vi "Absturz.vi"() -> ()   [LabVIEW 2020]
uses:
  <vilib>/xnet/xnet.llb/XNET Frame Type CAN.ctl
  <vilib>/xnet/xnet.llb/XNET Frame CAN.ctl
panel:
  out "I64":i64[](array[numeric])
  out "U64":u64[](array[numeric])
  in  "Numerisch":i32
  out "identifier":u32
  in  "Index":i32
  in  "CAN data 2":T1[](array[typedef])=[{"timestamp"=timestamp(0 s since 1904-01-01), "payload"=[0, 2, 3, 4, 5, 6, 7, 8], "identifier"=2, "type"=0, "extended?"=FALSE, "echo?"=FALSE}, {"timestamp"=timestamp(0 s since 1904-01-01), "payload"=[0, 1, 2, 3, 4, 5, 6, 7], "identifier"=3, "type"=0, "extended?"=FALSE, "echo?"=FALSE}] {"payload" format="%x"; "timestamp" format="%<%.7X\n%x>T"; "type" items=["CAN Data"=0, "CAN Remote"=1, "CAN Bus Error"=2, "CAN 2.0 Data"=8, "CAN FD Data"=16, "CAN FD+BRS Data"=24, "J1939 Data"=192, "Delay"=224, "Log Trigger"=225, "Start Trigger"=226]; "identifier" format="%x"}
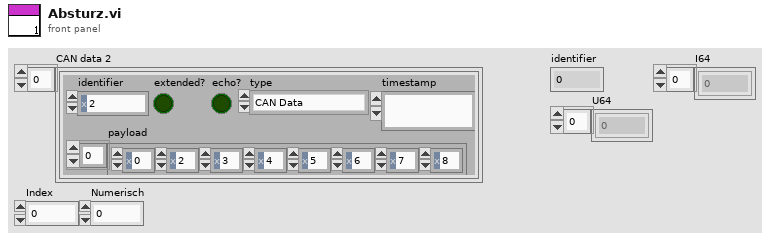
[diagram p1: front panel]
types:
  T1 = typedef "XNET Frame CAN.ctl" = cluster{"timestamp":timestamp, "payload":u8[], "identifier":u32, "type":T2, "extended?":bool, "echo?":bool}
  T2 = typedef "XNET Frame Type CAN.ctl" = u8
  T3 = enum16{"big-endian, network order", "native, host order", "little-endian"}
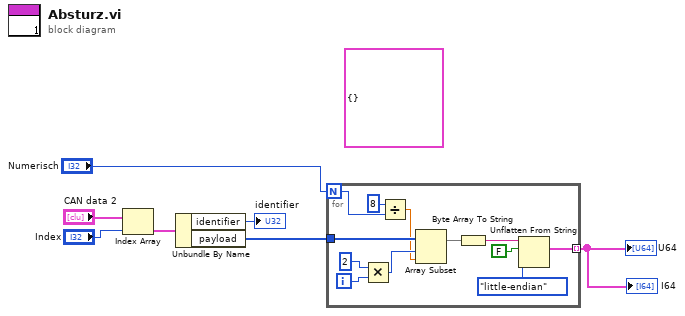
[diagram p0: block diagram]
diagram:
  (unwired) cluster{} {}
  n1 = Index Array(array="CAN data 2", index="Index") -> (element=w7:T1)
  n2 = Unbundle By Name(w7) -> ("identifier"=→"identifier":u32, "payload"=w6:u8[])
  n3 = for {
    N: "Numerisch" -> [w10]
    tunnel: w6 -> [w16]
    tunnel: [w11] -> w1 mode=indexing
    i -> [w19]
    n4 = Multiply(x=2, y=w19) -> (x*y=w17:i32)
    n5 = Divide(x=8, y=w10) -> (x/y=w8:dbl)
    n6 = Array Subset(array=w16, index=w17, length=w8) -> (w12:u8[])
    n7 = Byte Array To String(unsigned byte array=w12) -> (string=w13:string)
    n8 = Unflatten From String(binary string=w13, data includes array or string size? (T)=FALSE ("Enthält Array- oder String-Größe? (T)"), byte order (0:big-endian, network order)=T3."little-endian" ("Byte-Reihenfolge (0:Big-Endian, Netzwerkreihenfolge)")) -> (value=w11:cluster{})  [unwired: 2 in, 2 out]
  }
  "U64" <- w1
  "I64" <- w1
